vi "Read NET_WebProxy.vi"(8 "error in (no error)":errorcluster, 11 "WebProxy_NET in":refnum<class "WebProxy_NET.lvclass">) -> (0 "error out":errorcluster, 2 "NET_WebProxy":refnum<k24>, 3 "WebProxy_NET out":refnum<class "WebProxy_NET.lvclass">)   [LabVIEW 2018, in "HttpClient_NET.lvlib" / "WebProxy_NET.lvclass"]
uses:
  WebProxy_NET.lvclass
  WebProxy_NET.lvclass/WebProxy_NET.ctl
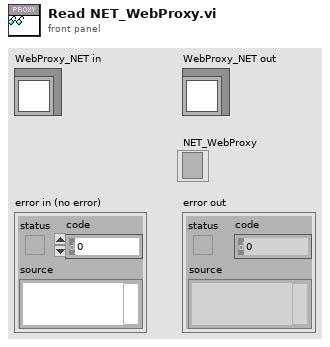
[diagram p1: front panel]
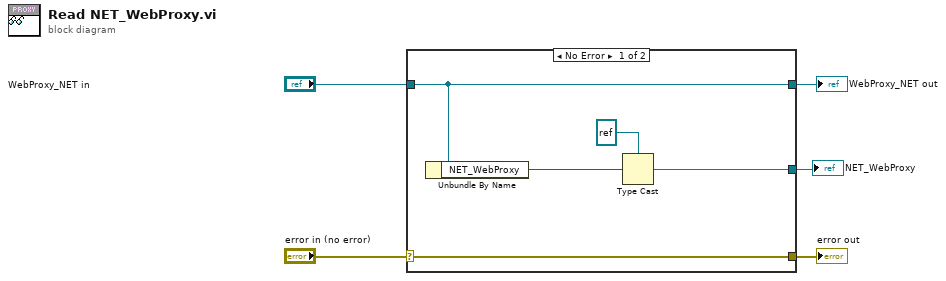
[diagram p0: block diagram]
diagram:
  n1 = case shown="No Error" "error in (no error)" {
    selector: "error in (no error)" -> [w10 w11]
    tunnel: [w10 w11] -> w4
    tunnel: [w9 w12] -> w2
    tunnel: "WebProxy_NET in" -> [w9 w12]
    tunnel: [w7 _] -> w1
    frame No Error {
      n2 = Unbundle By Name(w9) -> ("NET_WebProxy"=w8:i64)
      n3 = Type Cast(type=refnum<k24> refnum ("NET_WebProxy"), x=w8) -> (*(type *) &x=w7:refnum<k24>)
    }
    frame Error {
    }
  }
  "error out" <- w4
  "WebProxy_NET out" <- w2
  "NET_WebProxy" <- w1
